vi "PingTestMain.vi"() -> ()   [LabVIEW 2014]
uses:
  Lib/CEH.llb/EventMessage.ctl
  Lib/CEH.llb/InitializeEventHandling.vi
  Lib/CEH.llb/EventMemoryWrapperInitialization.vi
  Lib/CEH.llb/EnqueueEvent.vi
  Lib/CEH.llb/EventMemoryWrapperGetAll.vi
  Lib/CEH.llb/EnqueueAndDeleteError.vi
  Lib/CEH.llb/StopEventHandling.vi
panel:
  out "Last\nPing":bool
  out "Run":bool
  out "Pass/Fail":bool
  in  "GetEvents":bool
  out "EventMessages out":T1[](array[typedef])
  out "error out":errorcluster
  in  "IpAdress":string="192.168.101.2"
  in  "stop":bool
  in  "LogFileArchive: base path":path
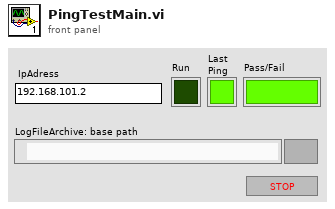
[diagram p1: front panel]
types:
  T1 = typedef "EventMessage.ctl" = cluster{"Identifier":enum16{"Event", "Error"}, "Data":variant}
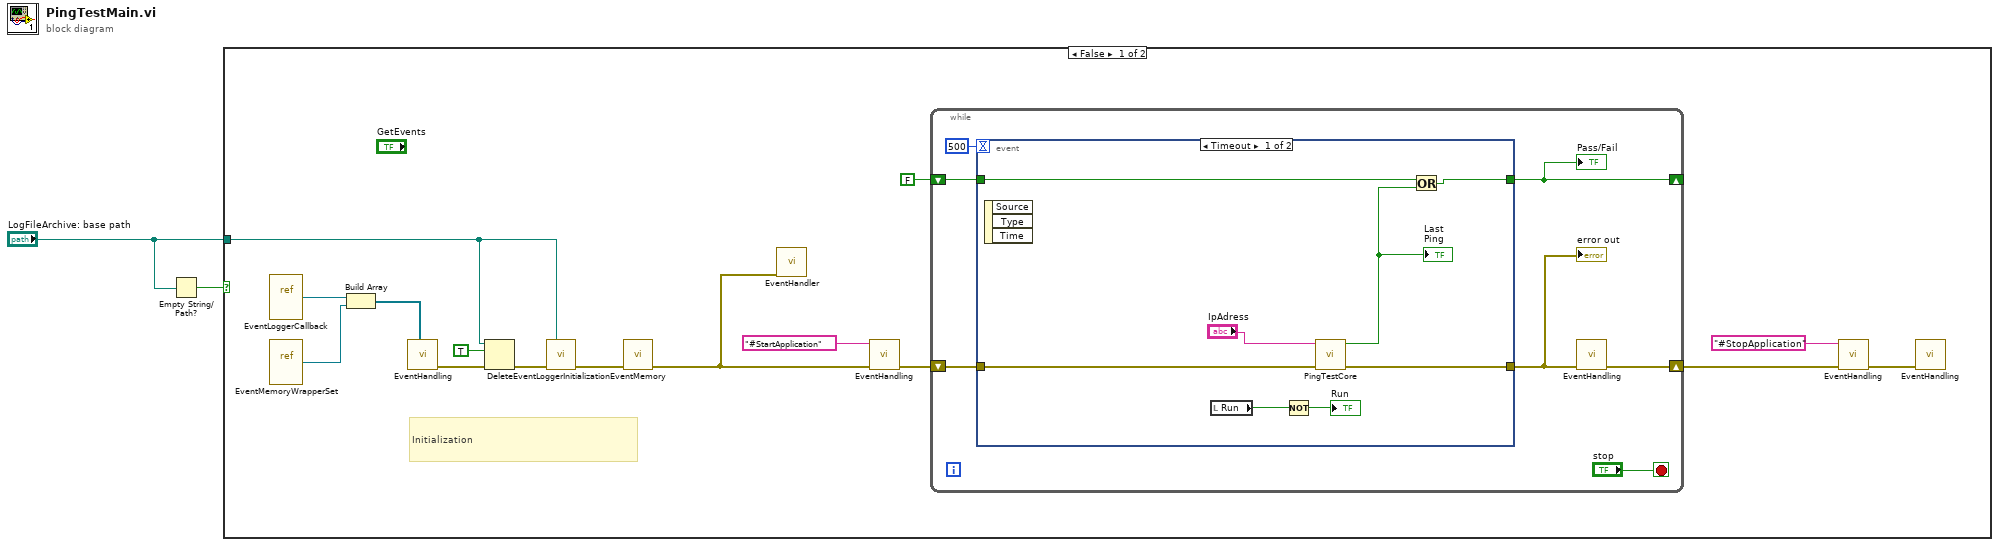
[diagram p0: block diagram]
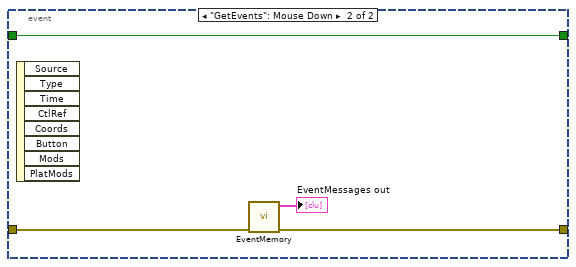
[diagram p2: hidden frame]
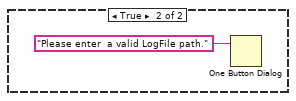
[diagram p3: hidden frame]
diagram:
  n1 = Empty String/Path?(string/path="LogFileArchive: base path") -> (empty?=w1:bool)
  n2 = case shown="False" w1 {
    tunnel: "LogFileArchive: base path" -> [w4 _]
    frame False {
      # "Initialization"
      n3 = vi-ref "EventLoggerCallback.vi"() -> (w13:refnum<vi>)
      n4 = vi-ref "EventMemoryWrapperSet.vi"() -> (w8:refnum<vi>)
      n5 = Build Array(w13, w8) -> (w12:refnum<vi>[])
      n6 = call-poly "EventHandling.vi"("OnEventCallbacks (VI Refs)"=w12) -> ("error out"=w6:errorcluster)  [unwired: 10 in]
      n7 = Delete(path (use dialog)=w4, entire hierarchy (F)=TRUE, error in=w6) -> (error out=w5:errorcluster)  [unwired: 2 in, 2 out]
      n8 = call "EventLoggerInitialization.vi"("LogFileArchive: base path"=w4, "error in"=w5) -> ("error out"=w17:errorcluster)  [unwired: 13 in]
      n9 = call-poly "EventMemory.vi"("error in"=w17) -> ("error out"=w10:errorcluster)  [unwired: 10 in]
      n10 = call "EventHandler.vi"("error in"=w10) -> ()  [unwired: 11 in]
      n11 = call-poly "EventHandling.vi"("error in"=w10, "EventIdentifyer"="#StartApplication" ("AdditionalData")) -> ("error out"=w9:errorcluster)  [unwired: 9 in]
      n12 = while {
        shift-right: [w22] -> w16
        shift-left: w9 -> [w24]
        shift-right: [w18] -> _
        shift-left: FALSE ("Failed?") -> [w19]
        stop <- "stop" stop-if-true
        n13 = event shown="[0] Timeout" {
          selector: _ -> [_ _]
          dyn-events: _ -> [_ _]
          timeout: 500 -> [_ _]
          tunnel: [w32 w34] -> w23
          tunnel: w24 -> [w31 w35]
          tunnel: [w28 w33] -> w18
          tunnel: w19 -> [w29 w33]
          event Timeout {
            n14 = event-data() -> ()  [unwired: 1 in, 3 out]
            n15 = local read "Run"() -> (w27:bool)
            n16 = Not(x=w27) -> (.not. x?=→"Run":bool)
            n17 = call "PingTestCore.vi"("error in (no error)"=w31, "IpAdress in"="IpAdress") -> ("error out"=w32:errorcluster, "Failed?"=w25:bool)  [unwired: 8 in]
            "Last\nPing" <- w25
            n18 = Or(x=w29, y=w25) -> (x .or. y?=w28:bool)
          }
          event "GetEvents": Mouse Down {
            n19 = event-data() -> ()  [unwired: 1 in, 8 out]
            n20 = call-poly "EventMemory.vi"("error in"=w35) -> ("error out"=w34:errorcluster, "EventMessages out"=→"EventMessages out":T1[])  [unwired: 9 in]
          }
        }
        "error out" <- w23
        "Pass/Fail" <- w18
        n21 = call-poly "EventHandling.vi"("error in"=w23) -> ("error out"=w22:errorcluster)  [unwired: 10 in]
      }
      n22 = call-poly "EventHandling.vi"("error in"=w16, "EventIdentifyer"="#StopApplication" ("AdditionalData")) -> ("error out"=w14:errorcluster)  [unwired: 9 in]
      n23 = call-poly "EventHandling.vi"("error in"=w14) -> ()  [unwired: 10 in, 1 out]
    }
    frame True {
      n24 = One Button Dialog(message="Please enter  a valid LogFile path.") -> ()  [unwired: 1 in, 1 out]
    }
  }
